vi "RydbergExpControl.vi"() -> ()   [LabVIEW 2013]
uses:
  rydberg_state_machine_states.ctl
  <userlib>/atmcd32d.llb/AcquisitionMode_mode typedef.ctl
  <userlib>/atmcd32d.llb/TriggerMode_mode typedef.ctl
  AndorCamera/camera_controls.ctl
  6704/6704_static_voltages_control.ctl
panel:
  in  "Path":path
  in  "base path":path
  out "error out":errorcluster
  in  "Tab Control":T1(tab)
  in  "Shutdown Experiment":bool
  in  "Start Experiment":bool
  in  "Instructions":T2(array[cluster])=[{"Instruct Data"=0, "Op Code"=0, "Flags"=[TRUE, FALSE, FALSE, FALSE, FALSE, FALSE, FALSE, FALSE, FALSE, FALSE, FALSE, FALSE, FALSE, FALSE, FALSE, FALSE, FALSE, FALSE, FALSE, FALSE, FALSE, FALSE, FALSE, FALSE], "Comments"="", "Time (s)"=0.1}, {"Instruct Data"=0, "Op Code"=0, "Flags"=[FALSE, FALSE, FALSE, FALSE, FALSE, FALSE, FALSE, FALSE, FALSE, FALSE, FALSE, FALSE, FALSE, FALSE, FALSE, FALSE, FALSE, FALSE, FALSE, FALSE, FALSE, FALSE, FALSE, FALSE], "Comments"="", "Time (s)"=0.1}, {"Instruct Data"=0, "Op Code"=0, "Flags"=[TRUE, FALSE, FALSE, FALSE, FALSE, FALSE, FALSE, FALSE, FALSE, FALSE, FALSE, FALSE, FALSE, FALSE, FALSE, FALSE, FALSE, FALSE, FALSE, FALSE, FALSE, FALSE, FALSE, FALSE], "Comments"="", "Time (s)"=0.1}, {"Instruct Data"=0, "Op Code"=6, "Flags"=[FALSE, FALSE, FALSE, FALSE, FALSE, FALSE, FALSE, FALSE, FALSE, FALSE, FALSE, FALSE, FALSE, FALSE, FALSE, FALSE, FALSE, FALSE, FALSE, FALSE, FALSE, FALSE, FALSE, FALSE], "Comments"="", "Time (s)"=0.1}] {"Time (s)" format="%.3p"; "Op Code" items=["Continue", "Stop", "Loop", "End Loop", "JSR", "RTS", "Branch", "Long Delay", "Wait"]}
  out "Camera Information":T3 {"VS Speed (us)" format="%.2f"}
  in  "Acquisition Parameters":T4={"Acquisition Mode"=enum."Single Scan", "Trigger Mode"=enum."Internal", "Frame \nTransfer"=FALSE, "Exposure Time (s)"=0.0, "Accumulation Cycle Time (s)"=0.0, "# Accumulations"=1, "# Kinetics"=1, "Kinetic Cycle Time (s)"=0.0} {"Kinetic Cycle Time (s)" format="%.4f"; "# Kinetics" min=1; "# Accumulations" min=1; "Accumulation Cycle Time (s)" format="%.4f"; "Exposure Time (s)" format="%.4f"}
  out "Calcualted Times":T7 {"Kinetic" format="%.4f"; "Accumulate" format="%.4f"; "Exposure" format="%.4f"}
  in  "Red MOT 87 Inputs":T8 {"Waveform Parameters"."Degree" min=1}
  in  "6704 Static Voltage Settings":T9
  out "Andor Initialization Error Codes":T10
  out "Acq. Error Codes":T11
  in  "File To Load":path
  out "Tree":string(tree)
  # "1"
  # "2"
  # "3"
  # "4"
  # "5"
  # "6"
  # "7"
  # "8"
  # "9"
  # "10"
  # "11"
  # "12"
  # "13"
  # "14"
  # "15"
  # "16"
  # "17"
  # "18"
  # "19"
  # "20"
  # "21"
  # "22"
  # "23"
  # "24"
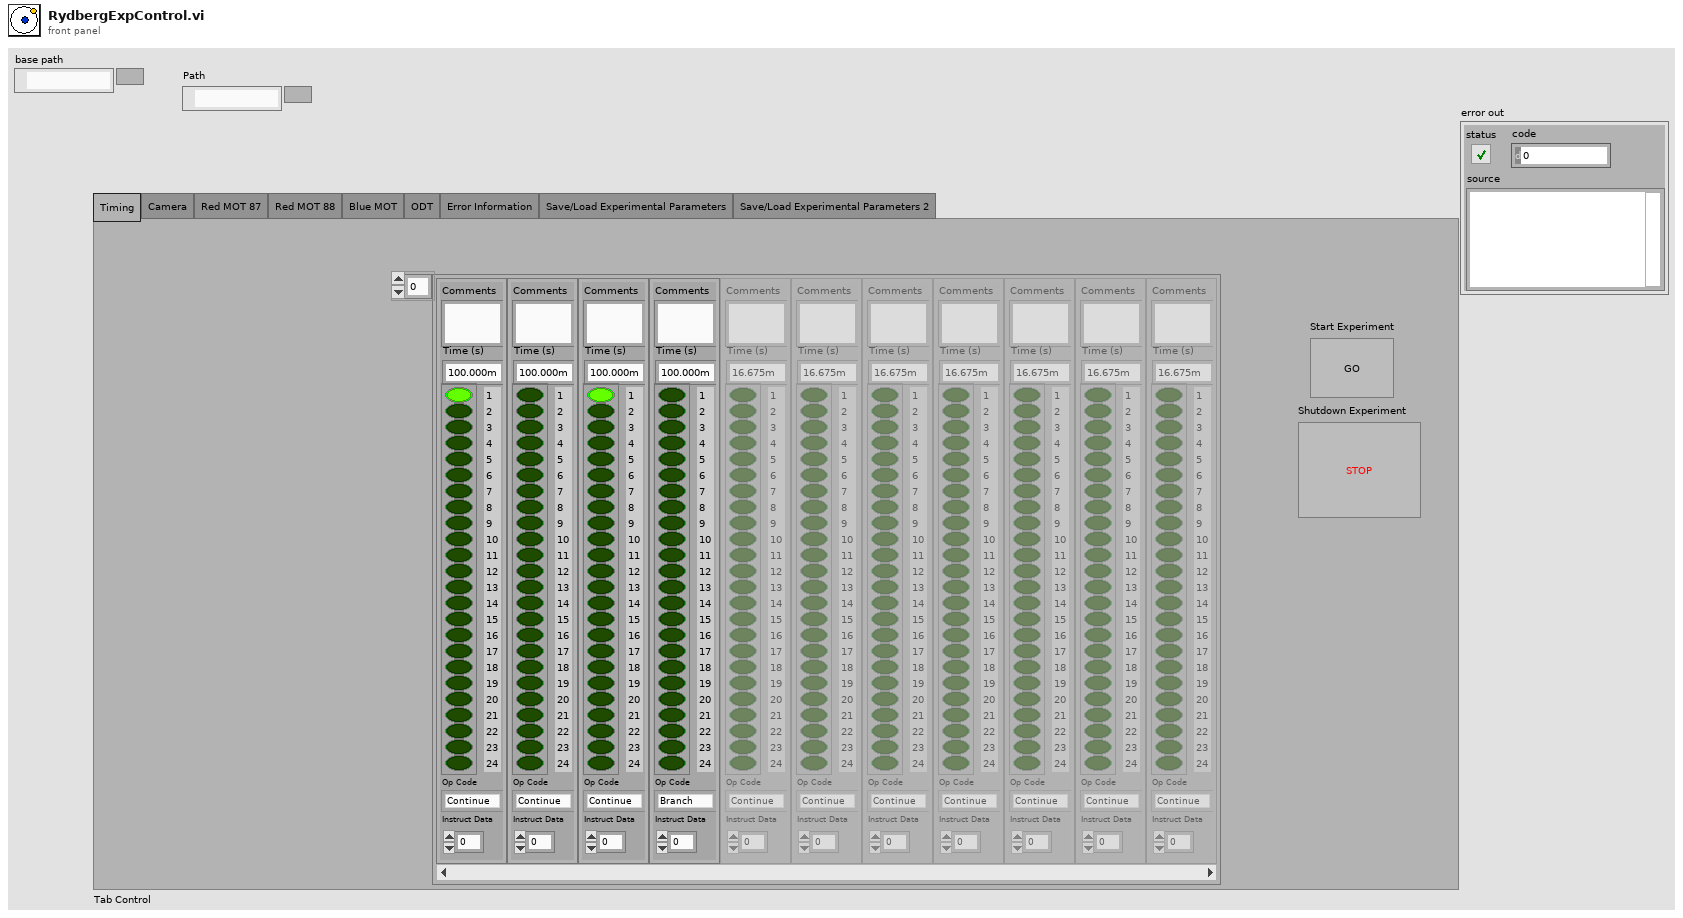
[diagram p1: front panel]
types:
  T1 = enum32{"Timing", "Camera", "Red MOT 87", "Red MOT 88", "Blue MOT", "ODT", "Error Information", "Save/Load Experimental Parameters", "Save/Load Experimental Parameters 2"}
  T2 = cluster{"Instruct Data":i32, "Op Code":i32, "Flags":bool[], "Comments":string, "Time (s)":dbl}[]
  T3 = cluster{"xpixels":i32, "ypixels":i32, "# VS Speeds":i32, "VS Speed (us)":sgl, "Temperature Stable":bool, "Temperature (C)":i32}
  T4 = typedef "camera_controls.ctl" = cluster{"Acquisition Mode":T5, "Trigger Mode":T6, "Frame \nTransfer":bool, "Exposure Time (s)":sgl, "Accumulation Cycle Time (s)":sgl, "# Accumulations":i32, "# Kinetics":i32, "Kinetic Cycle Time (s)":sgl}
  T5 = typedef "AcquisitionMode_mode typedef.ctl" = enum16{"Reserved (0)", "Single Scan", "Accumulate", "Kinetics", "Fast Kinetics", "Run Till Abort", "Reserved (6)", "Reserved (7)", "Reserved (8)", "Time Delayed Integration"}
  T6 = typedef "TriggerMode_mode typedef.ctl" = enum16{"Internal", "External", "N/A (2)", "N/A (3)", "N/A (4)", "N/A (5)", "External Start", "External Exposure (Bulb)", "N/A (8)", "External FVB EM", "Software", "N/A (11)", "External Charge Shifting"}
  T7 = cluster{"Exposure":sgl, "Accumulate":sgl, "Kinetic":sgl}
  T8 = cluster{"Active Device":string, "Active Channels":bool[], "Waveform Parameters":cluster{"Functional Form":enum16{"Polynomial", "Exponential"}, "Start Voltage":dbl, "End Voltage":dbl, "Time":dbl, "Degree":i8, "Sample Rate":dbl}[][], "Active Phases":bool[], "Phase Times":dbl[], "Trigger Channel":tag}
  T9 = typedef "6704_static_voltages_control.ctl" = cluster{"Device Name":string, "Voltages":dbl[]}
  T10 = cluster{"Initalize Error Code":u32, "GetDetector Error Code":u32, "Get#VSSpeeds Error Code":u32, "Set VS Speed Error":u32, "CoolerOn Error Code":u32, "GetTemperature Error Code":u32, "Shutdown Error Code":u32}
  T11 = cluster{"Set Acq. Mode Error":u32, "Set Trigger Mode Error":u32, "Set FT Error Code":u32, "Set Exposure Time Error Code":u32, "Set Accum Time Error":u32, "Set # Accum Error":u32, "Set # Kinetics Error":u32, "SetKinCycleTime Error":u32}
  T12 = typedef "rydberg_state_machine_states.ctl" = enum16{"Initialize", "Idle", "Go", "Load Experiment", "Shutdown"}
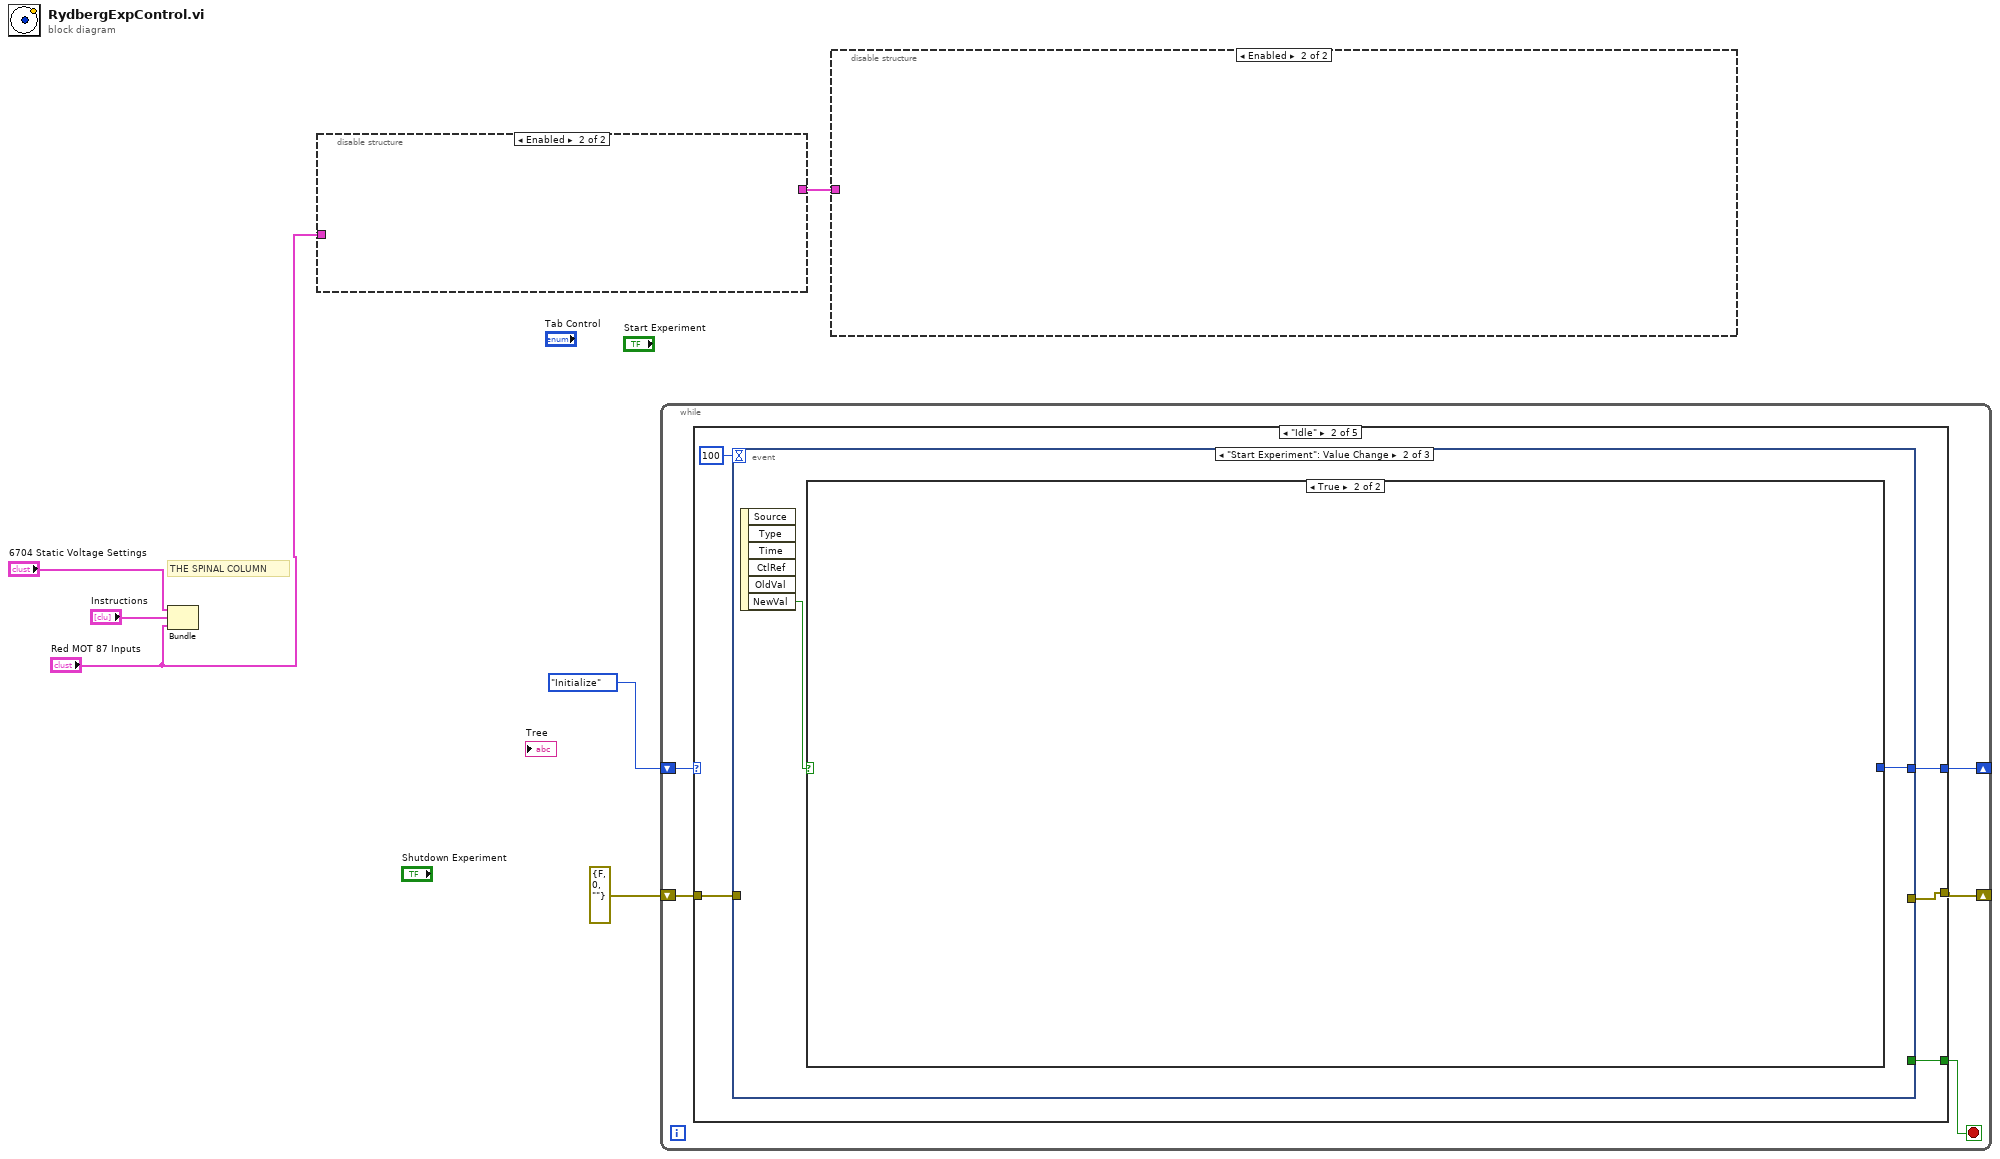
[diagram p0: block diagram]
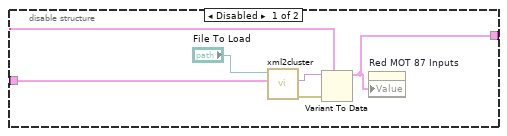
[diagram p2: hidden frame]
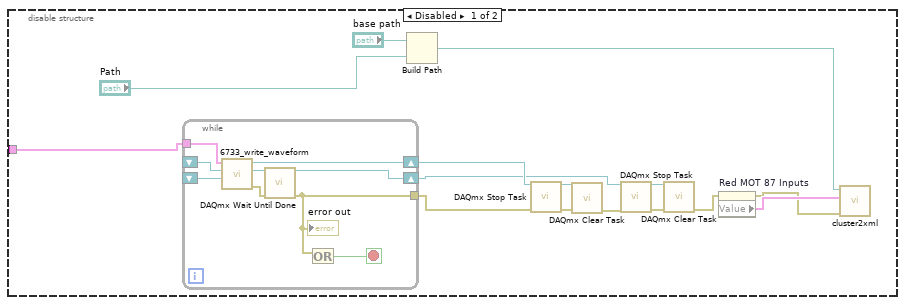
[diagram p3: hidden frame]
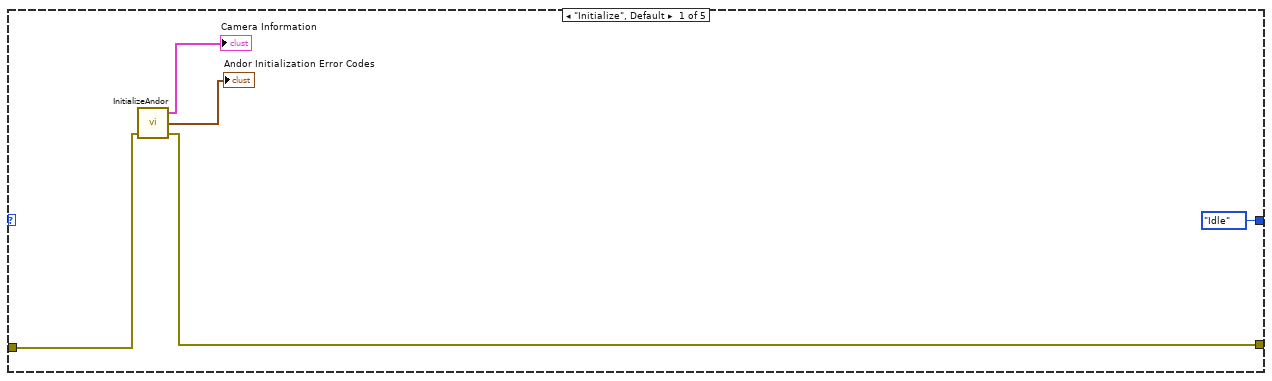
[diagram p4: hidden frame]
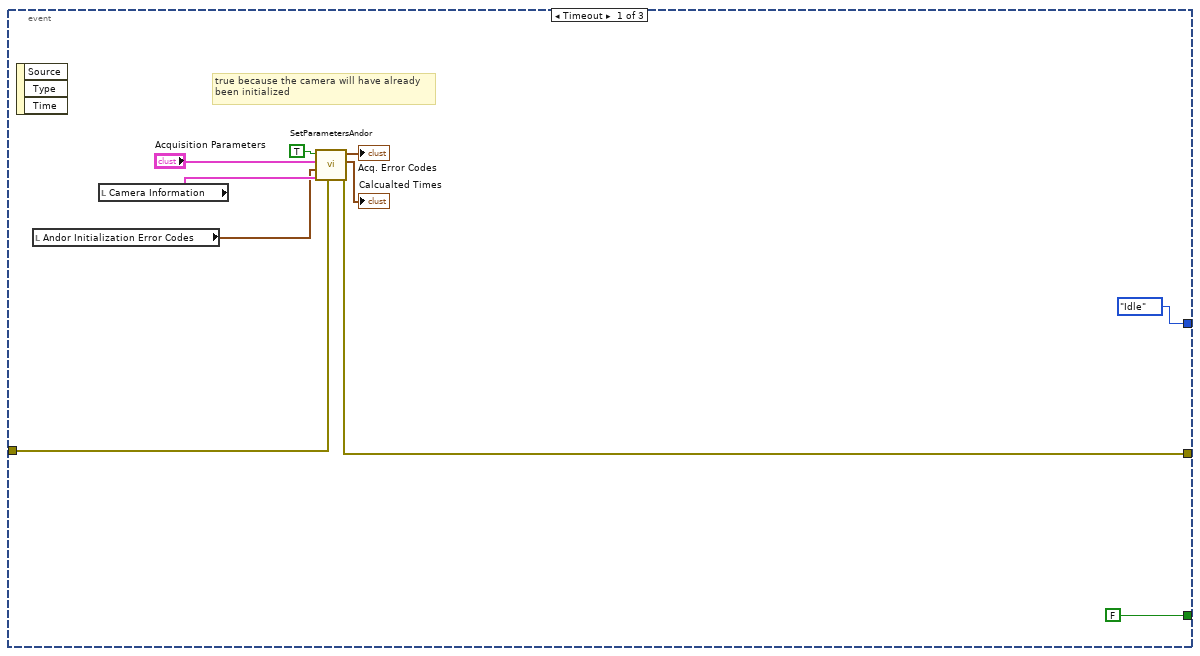
[diagram p5: hidden frame]
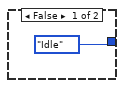
[diagram p6: hidden frame]
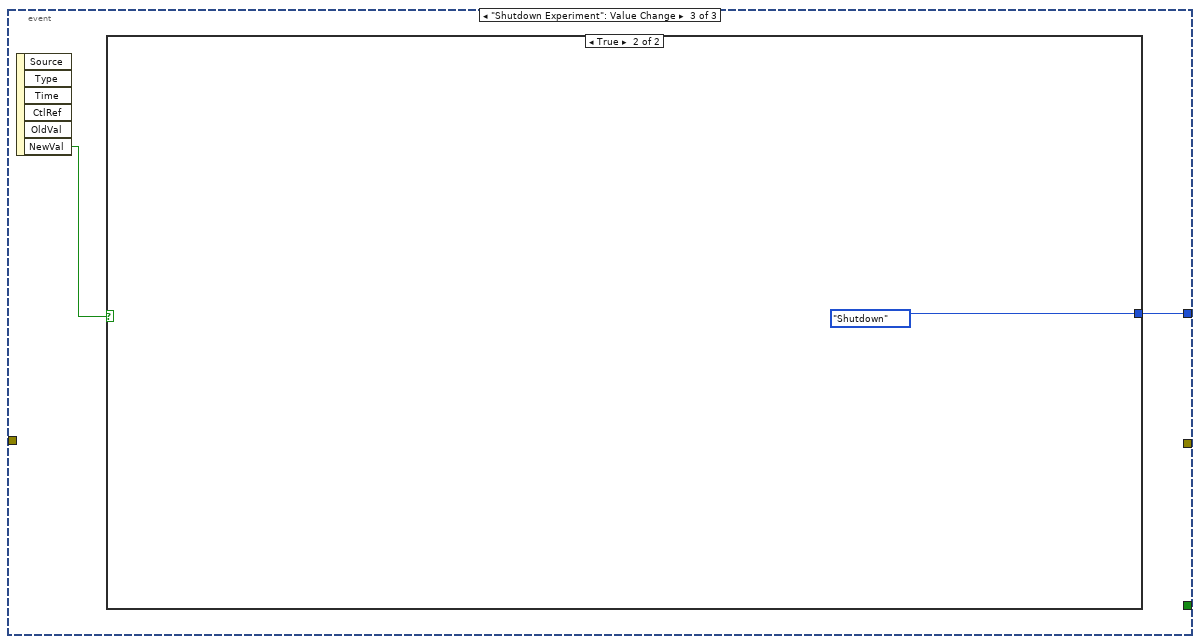
[diagram p7: hidden frame]
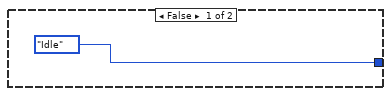
[diagram p8: hidden frame]
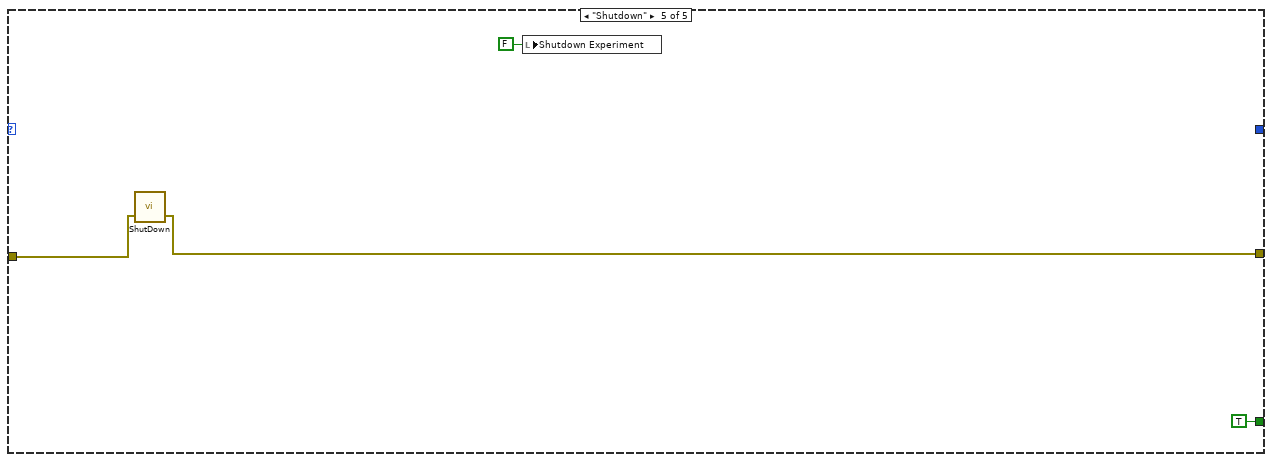
[diagram p11: hidden frame]
diagram:
  # "THE SPINAL COLUMN"
  n1 = Bundle("6704 Static Voltage Settings"="6704 Static Voltage Settings", "Instructions"="Instructions", "Red MOT 87 Inputs"="Red MOT 87 Inputs") -> ()  [unwired: 1 in, 1 out]
  n2 = disable-structure shown="Enabled" {
    disable-tunnel: [w9 _] -> w6
    disable-tunnel: "Red MOT 87 Inputs" -> [w7 _]
    frame Disabled {
      n3 = call "xml2cluster.vi"("TypeDesc"=w7, "XML File Path"="File To Load") -> ("error out"=w11:errorcluster, "data"=w10:variant)  [unwired: 7 in, 1 out]
      n4 = Variant To Data(error in=w11, type=w7, Variant=w10) -> (data=w9:T8)  [unwired: 1 out]
      n5 = property on="Red MOT 87 Inputs" class="Clust (strict)"("Value"=w9) -> ()  [unwired: 2 in, 2 out]
    }
    frame Enabled {
    }
  }
  n6 = while {
    shift-right: [w13] -> _
    shift-left: rydberg_state_machine_states."Initialize" -> [w16]
    shift-right: [w14] -> _
    shift-left: errorcluster {"status"=FALSE, "code"=0, "source"=""} ("error constant") -> [w15]
    stop <- w12 stop-if-true
    n7 = case shown="\"Idle\"" w16 {
      tunnel: w15 -> [w21 w26 _ _ w47]
      tunnel: [w18 w22 _ _ w46] -> w14
      tunnel: [rydberg_state_machine_states."Idle" w24 _ _ _] -> w13
      tunnel: [_ w23 _ _ TRUE] -> w12
      frame "Initialize", Default {
        n8 = call "InitializeAndor.vi"("Error In"=w21) -> ("error out"=w18:errorcluster, "Andor Initialization Error Codes"=→"Andor Initialization Error Codes":T10, "Camera Information"=→"Camera Information":T3)  [unwired: 2 in]
      }
      frame "Idle" {
        n9 = event shown="[1] \"Start Experiment\": Value Change" {
          selector: _ -> [_ _ _]
          dyn-events: _ -> [_ _ _]
          timeout: 100 -> [_ _ _]
          tunnel: w26 -> [w30 _ _]
          tunnel: [rydberg_state_machine_states."Idle" w37 w40] -> w24
          tunnel: [FALSE _ _] -> w23
          tunnel: [w29 _ _] -> w22
          event Timeout {
            # "true because the camera will have already\nbeen initialized"
            n10 = event-data() -> ()  [unwired: 1 in, 3 out]
            n11 = local read "Andor Initialization Error Codes"() -> (w28:T10)
            n12 = local read "Camera Information"() -> (w32:T3)
            n13 = call "SetParametersAndor.vi"("Error In"=w30, "Camera Information"=w32, "Andor Initialization Error Codes"=w28, "Acquisition Parameters"="Acquisition Parameters", "Pre Initialized?"=TRUE) -> ("error out"=w29:errorcluster, "Calcualted Times"=→"Calcualted Times":T7, "Acq. Error Codes"=→"Acq. Error Codes":T11)  [unwired: 4 in]
          }
          event "Start Experiment": Value Change {
            n14 = event-data() -> ("NewVal"=w38:bool)  [unwired: 1 in, 5 out]
            n15 = case shown="True" w38 {
              tunnel: [rydberg_state_machine_states."Idle" _] -> w37
              frame False {
              }
              frame True {
              }
            }
          }
          event "Shutdown Experiment": Value Change {
            n16 = event-data() -> ("NewVal"=w41:bool)  [unwired: 1 in, 5 out]
            n17 = case shown="True" w41 {
              tunnel: [rydberg_state_machine_states."Idle" rydberg_state_machine_states."Shutdown"] -> w40
              frame False {
              }
              frame True {
              }
            }
          }
        }
      }
      frame "Go" {
      }
      frame "Load Experiment" {
      }
      frame "Shutdown" {
        n18 = call <userlib>:"ShutDown.vi"("error in (no error)"=w47) -> ("error out"=w46:errorcluster)  [unwired: 1 in, 1 out]
        n19 = local write "Shutdown Experiment"(FALSE ("Shutdown Experiment")) -> ()
      }
    }
  }
  n20 = disable-structure shown="Enabled" {
    disable-tunnel: w6 -> [w54 _]
    frame Disabled {
      n21 = while {
        tunnel: w54 -> [w63]
        shift-right: [w71] -> w57
        shift-left: _ -> [w70]
        shift-right: [w66] -> w56
        shift-left: _ -> [w69]
        tunnel: [w64] -> w55
        stop <- w68 stop-if-true
        n22 = call "6733_write_waveform.vi"("Control Task In"=w69, "Waveform Task In"=w70, "Inputs"=w63) -> ("error out"=w65:errorcluster, "counter task out"=w67:refnum<k21>, "waveform task out"=w71:refnum<k21>)  [unwired: 6 in]
        n23 = call <vilib>:"DAQmx Wait Until Done.vi"("task/channels in"=w67, "error in"=w65) -> ("task out"=w66:refnum<k21>, "error out"=w64:errorcluster)  [unwired: 12 in]
        "error out" <- w64
        n24 = Or(x=w64) -> (y=w72:errorcluster, x .or. y?=w68:bool)
      }
      n25 = Build Path(base path="base path", name or relative path="Path") -> (appended path=w48:path)
      n26 = call <vilib>:"DAQmx Stop Task.vi"("task/channels in"=w57, "error in"=w55) -> ("task out"=w62:refnum<k21>, "error out"=w61:errorcluster)  [unwired: 12 in]
      n27 = call <vilib>:"DAQmx Clear Task.vi"("task in"=w62, "error in"=w61) -> ("error out"=w58:errorcluster)  [unwired: 13 in]
      n28 = call <vilib>:"DAQmx Stop Task.vi"("task/channels in"=w56, "error in"=w58) -> ("task out"=w60:refnum<k21>, "error out"=w59:errorcluster)  [unwired: 12 in]
      n29 = call <vilib>:"DAQmx Clear Task.vi"("task in"=w60, "error in"=w59) -> ("error out"=w53:errorcluster)  [unwired: 13 in]
      n30 = property on="Red MOT 87 Inputs" class="Clust (strict)"(error in=w53) -> (error out=w51:errorcluster, "Value"=w52:T8)  [unwired: 1 in, 1 out]
      n31 = call "cluster2xml.vi"("error in"=w51, "Variant"=w52, "XML File Path"=w48) -> ()  [unwired: 8 in, 1 out]
    }
    frame Enabled {
    }
  }
